vi "2x2 binning.vi"() -> ()   [LabVIEW 2012, in "DAQCascade512II.lvclass"]
uses:
  DAQCascade512II.lvclass
  DAQCascade512II.lvclass/DAQCascade512II.ctl
panel:
  out "2x2 binning":bool
  out "error out":errorcluster
  in  "error in":errorcluster
  out "DAQCascade512II out":refnum<class "DAQCascade512II.lvclass">
  in  "DAQCascade512II in":refnum<class "DAQCascade512II.lvclass">
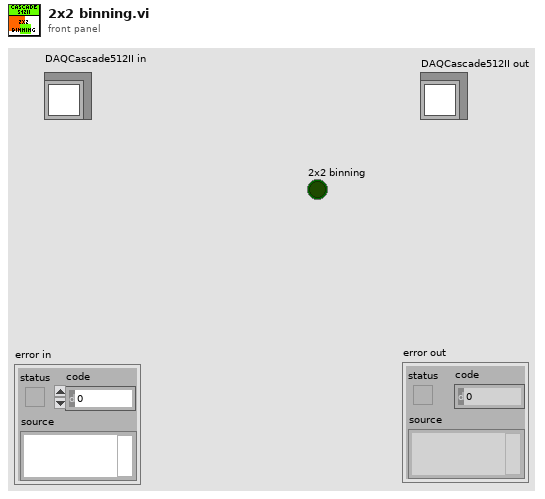
[diagram p1: front panel]
types:
  T1 = cluster{"X start":u32, "X end":u32, "X Binning/Grouping":u32, "Y start":u32, "Y end":u32, "Y Binning/Grouping":u32}
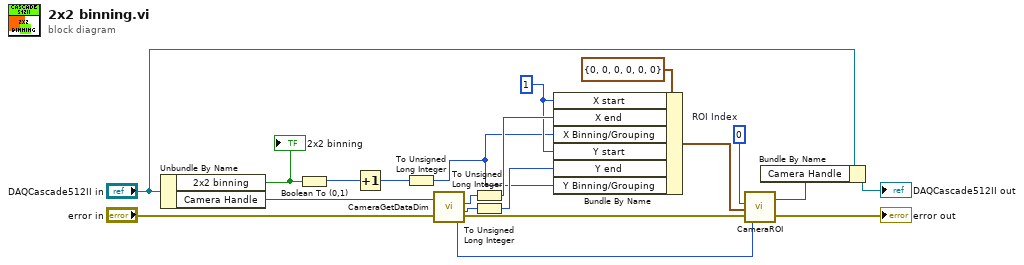
[diagram p0: block diagram]
diagram:
  w14 = u32 0  # ROI Index
  w15 = u32 1
  n1 = Unbundle By Name("DAQCascade512II in") -> ("2x2 binning"=w7:bool, "Camera Handle"=w10:u32)
  "2x2 binning" <- w7
  n2 = Boolean To (0,1)(Boolean=w7) -> (0, 1=w6:i16)
  n3 = Increment(x=w6) -> (x+1=w5:i16)
  n4 = To Unsigned Long Integer(number=w5) -> (unsigned 32bit integer=w4:u32)
  n5 = call <userlib>:"CameraGetDataDim.vi"("Camera Handle"=w10, "error in"="error in") -> ("Camera Handle"=w11:u32, "Xdim"=w16:u32, "Ydim"=w18:u32, "error out"=w12:errorcluster)
  n6 = To Unsigned Long Integer(number=w16) -> (unsigned 32bit integer=w17:u32)
  n7 = To Unsigned Long Integer(number=w18) -> (unsigned 32bit integer=w19:u32)
  n8 = Bundle By Name(cluster=T1 {"X start"=0, "X end"=0, "X Binning/Grouping"=0, "Y start"=0, "Y end"=0, "Y Binning/Grouping"=0} ("ROI Params"), "X start"=w15, "X end"=w17, "X Binning/Grouping"=w4, "Y start"=w15, "Y end"=w19, "Y Binning/Grouping"=w4) -> (w20:T1)
  n9 = call <userlib>:"CameraROI.vi"("error in"=w12, "ROI Params"=w20, "ROI Index"=w14, "Camera Handle"=w11) -> ("error out"=→"error out":errorcluster, "Camera Handle"=w2:u32)
  n10 = Bundle By Name(cluster="DAQCascade512II in", "Camera Handle"=w2) -> (→"DAQCascade512II out":refnum<class "DAQCascade512II.lvclass">)
